vi "MAIN PROGRAM.vi"() -> ()   [LabVIEW 2021]
uses:
  ctlTrialState.ctl
  ctlProtocol.ctl
  ctlProtocolSubID.ctl
  ctlBlockOrder.ctl
  ctrBlockCondition.ctl
  ctrLED_R2L.ctl
  ctrCMCondition.ctl
  ctlSeqFNs.ctl
  ctrBlockInfo.ctl
  ctlBlockInfoSet.ctl
  ctlPkgMain.ctl
  ctlSeqFNs_SubVI PhaseSpace.ctl
  ctlSeqFNs_SubVI ATI.ctl
  ctrOWLMarker.ctl
  ctldistance2plane.ctl
  ctrTrialInfo.ctl
  ctlRecording.ctl
  <vilib>/Analysis/coordinate.llb/Euler Rotation Order.ctl
  <vilib>/DAQmx/write.llb/DAQmx Write (Digital 1D U8 1Chan NSamp).vi
  <vilib>/Analysis/baseanly.llb/A x Vector.vi
  <vilib>/Analysis/baseanly.llb/Real A x B.vi
  <vilib>/Analysis/_algsub.llb/Real Vector Norm.vi
  GLOBAL -MAIN.vi
  <vilib>/DAQmx/miscellaneous.llb/DAQmx Fill In Error Info.vi
  <vilib>/Analysis/Matrix/Numeric/Conversions/Array To Matrix - RA2.vi
  <vilib>/Analysis/Matrix/Numeric/Conversions/Matrix To Array - RM.vi
  <vilib>/Analysis/Matrix/Numeric/Conversions/Array To Matrix - RA.vi
  <vilib>/Analysis/NI_AALBase.lvlib
  <vilib>/Analysis/Matrix/NI_Matrix.lvlib
  <vilib>/Analysis/NI_AALPro.lvlib
panel:
  out "|FM| (N)":dbl format="%#_2g"
  out "|FG| (N)":dbl format="%#_2g"
  out "FM":dbl[](array[numeric]) format="%#_2g"
  out "FG":dbl[](array[numeric]) format="%#.2g"
  out "Roll (deg)":dbl(graph)
  out "Meter":dbl(knob) scale=-15.0..15.0 scale format="%#_2g"
  in  "Time Target (s)":i64=5000
  out "My":dbl
  out "Mx":dbl
  out "friction test?":bool
  out "max roll":dbl
  out "max height":dbl
  in  "BlockInfoSet":T1 {"Trial#-1 in block" min=0 max=11 step=1}
  out "BlockInfoConfig":T2={"block #"=0, "block cond"=enum."RHP", "Trial # in block"=0}
  in  "Subject ID":T4
  out "Current Trial #":i32
  out "Current & finished":T2={"block #"=0, "block cond"=enum."RHP", "Trial # in block"=0}
  out "SYS STATE":T5=enum."INITIALIZE Sub"
  out "CM cond":T6
  out "dCOP (mm)":dbl format="%#_2g"
  out "dCOP cond":T7 items=["all off"=0, "all on"=63, "0 mm"=1, "+8.84 mm"=2, "+15.76 mm"=3, "+22.68 mm"=4, "+29.60 mm"=5, "+36.52 mm"=6, "+43.44 mm"=7, "+50.36 mm"=8, "+57.28 mm"=9, "+64.20 mm"=10, "-8.84 mm"=11, "-15.76 mm"=12, "-22.68 mm"=13, "-29.60 mm"=14, "-36.52 mm"=15, "-43.44 mm"=16, "-50.36 mm"=17, "-57.28 mm"=18, "-64.20 mm"=19]
  out "resultant force":cluster{dbl}(graph)
  out "h (mm)":dbl(graph)
  in  "RepeatTrial":bool
  in  "Recording?":bool=TRUE
  in  "hold criterion (mm)":dbl=50.0 min=0.0 max=500.0 step=1.0
  in  "Path":path=path "C:/Users/NCML/Desktop/GraspEMG/data"
  in  "Bias":bool
  out "ATI":cluster{dbl[][]}[](array[cluster]) {"?" format="%#.2f"}
  out "Protocol":T8={"Subject ID"=enum."sub-09", "Block order"=[enum."famDrop", enum."preDrop", enum."famTask", enum."UL", enum."UR", enum."RHP", enum."LHP", enum."RHD", enum."RLD", enum."LLD", enum."LHD", enum."pstDrop"]}
  out "state":T10
  in  "STOP":bool
  in  "Ready":bool
  out "Date & Time":timestamp format="%<%.3X %x>T"
  # "Recieves data from both SubVIs"
  # "(CCW -; CW +)"
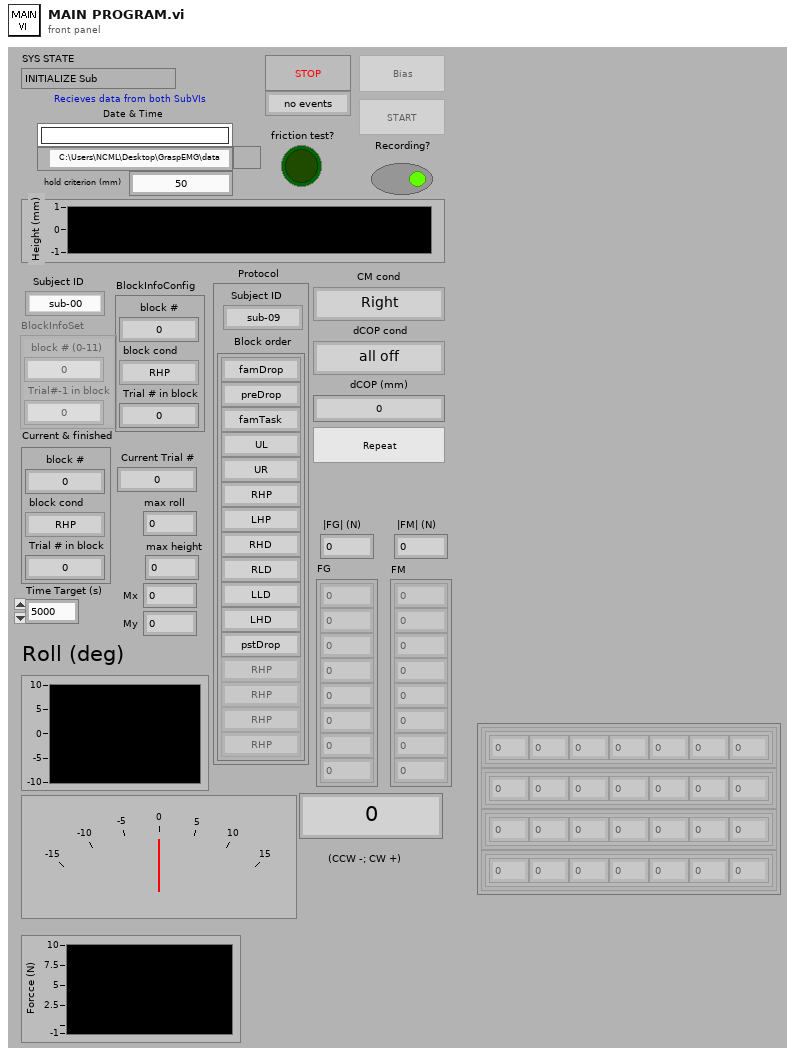
[diagram p1: front panel]
types:
  T1 = typedef "ctlBlockInfoSet.ctl" = cluster{"block # (0-11)":i32, "Trial#-1 in block":i32}
  T2 = typedef "ctrBlockInfo.ctl" = cluster{"block #":i32, "block cond":T3, "Trial # in block":i32}
  T3 = typedef "ctrBlockCondition.ctl" = enum16{"famDrop", "preDrop", "famTask", "RHP", "RLD", "RHD", "LHP", "LLD", "LHD", "UR", "UL", "pstDrop"}
  T4 = typedef "ctlProtocolSubID.ctl" = enum16{"sub-00", "sub-01", "sub-02", "sub-03", "sub-04", "sub-05", "sub-06", "sub-07", "sub-08", "sub-09", "sub-10", "sub-11", "sub-12", "sub-13", "sub-14", "sub-15", "sub-16", "sub-17", "sub-18", "sub-19", "sub-20", "sub-21", "sub-22", "sub-23", "sub-24", "sub-25", "sub-26", "sub-27", "sub-28", "sub-29", "sub-30", "sub-31", "sub-32", "sub-33", "sub-34", "sub-35", "sub-36", "sub-37", "sub-38", "sub-39", "sub-40"}
  T5 = typedef "ctlSeqFNs.ctl" = enum16{"INITIALIZE MAIN", "UpdateProtocol", "UpdateBlockInfo", "UpdatePath", "INITIALIZE Sub", "IDLE", "Bias", "Ready", "RepeatTrial", "Events", "Get PS bias", "Get PhaseSpace", "Get ATI", "Finish", "End PhaseSpace", "End ATI", "ERROR", "EXIT"}
  T6 = typedef "ctrCMCondition.ctl" = enum16{"Right", "Center", "Left"}
  T7 = typedef "ctrLED_R2L.ctl" = u16
  T8 = typedef "ctlProtocol.ctl" = cluster{"Subject ID":T4, "Block order":T9}
  T9 = typedef "ctlBlockOrder.ctl" = T3[]
  T10 = typedef "ctlTrialState.ctl" = enum16{"no events", "ready", "start", "hold", "stop", "end"}
  T11 = typedef "ctlPkgMain.ctl" = cluster{"VIRefNm ":refnum<vi>, "PhaseSpace":refnum<queue>, "ATI":refnum<queue>, "Handle Height":dbl, "Results":cluster{"Kc":string, "Cfg":dbl[]}, "CurrPath":path, "state":T10, "tick ini":i64, "Protocol":T8, "PhaseSpace end?":bool, "ATI end?":bool, "Markers":T12[], "ATI Data":cluster{dbl[][]}[], "d2plane":T13, "data Path":path, "PreTrialInfo":T14, "tdms data":refnum<k34>, "Recording?":bool, "dCOP cond":T7, "TrialInfo":T14, "Handle Tilt":dbl, "maxheight":dbl, "maxroll":dbl, "friction test?":bool, "Trigger Task":refnum<k21>}
  T12 = typedef "ctrOWLMarker.ctl" = cluster{"id":i32, "frame":i32, "x":sgl, "y":sgl, "z":sgl, "cond":sgl, "flag":u32}
  T13 = typedef "ctldistance2plane.ctl" = cluster{"frame":dbl[][]}
  T14 = typedef "ctrTrialInfo.ctl" = cluster{"BlockInfo":T2, "Trial #":i32}
  T15 = enum8{"Enabled", "Disabled", "Disabled and Grayed Out"}
  T16 = enum16{"ALIGN -CENTER", "ALIGN -TOP LEFT", "ALIGN -AS IS", "ALIGN -CUSTOM"}
  T17 = enum16{"open", "open or create", "create or replace", "create", "open (read-only)"}
  T18 = typedef "ctlSeqFNs_SubVI ATI.ctl" = enum16{"INITIALIZE", "SET HANDLE", "IDLE", "READY", "SEND2MAIN", "CALIB Load", "BIAS", "TRIGGER", "END", "ERROR", "EXIT"}
  T19 = typedef "ctlSeqFNs_SubVI PhaseSpace.ctl" = enum16{"INITIALIZE", "IDLE", "BIAS", "READY", "SEND2MAIN", "LOG2TDMS", "TRIGGER", "END", "ERROR", "EXIT"}
  T20 = typedef "ctlRecording.ctl" = cluster{"recording?":bool, "tdms file":refnum<k34>}
  T21 = typedef "NI_AALPro.lvlib/Euler Rotation Order.ctl" = u16
  T22 = typedef "NI_Matrix.lvlib/RealMatrix.ctl" = dbl[][]
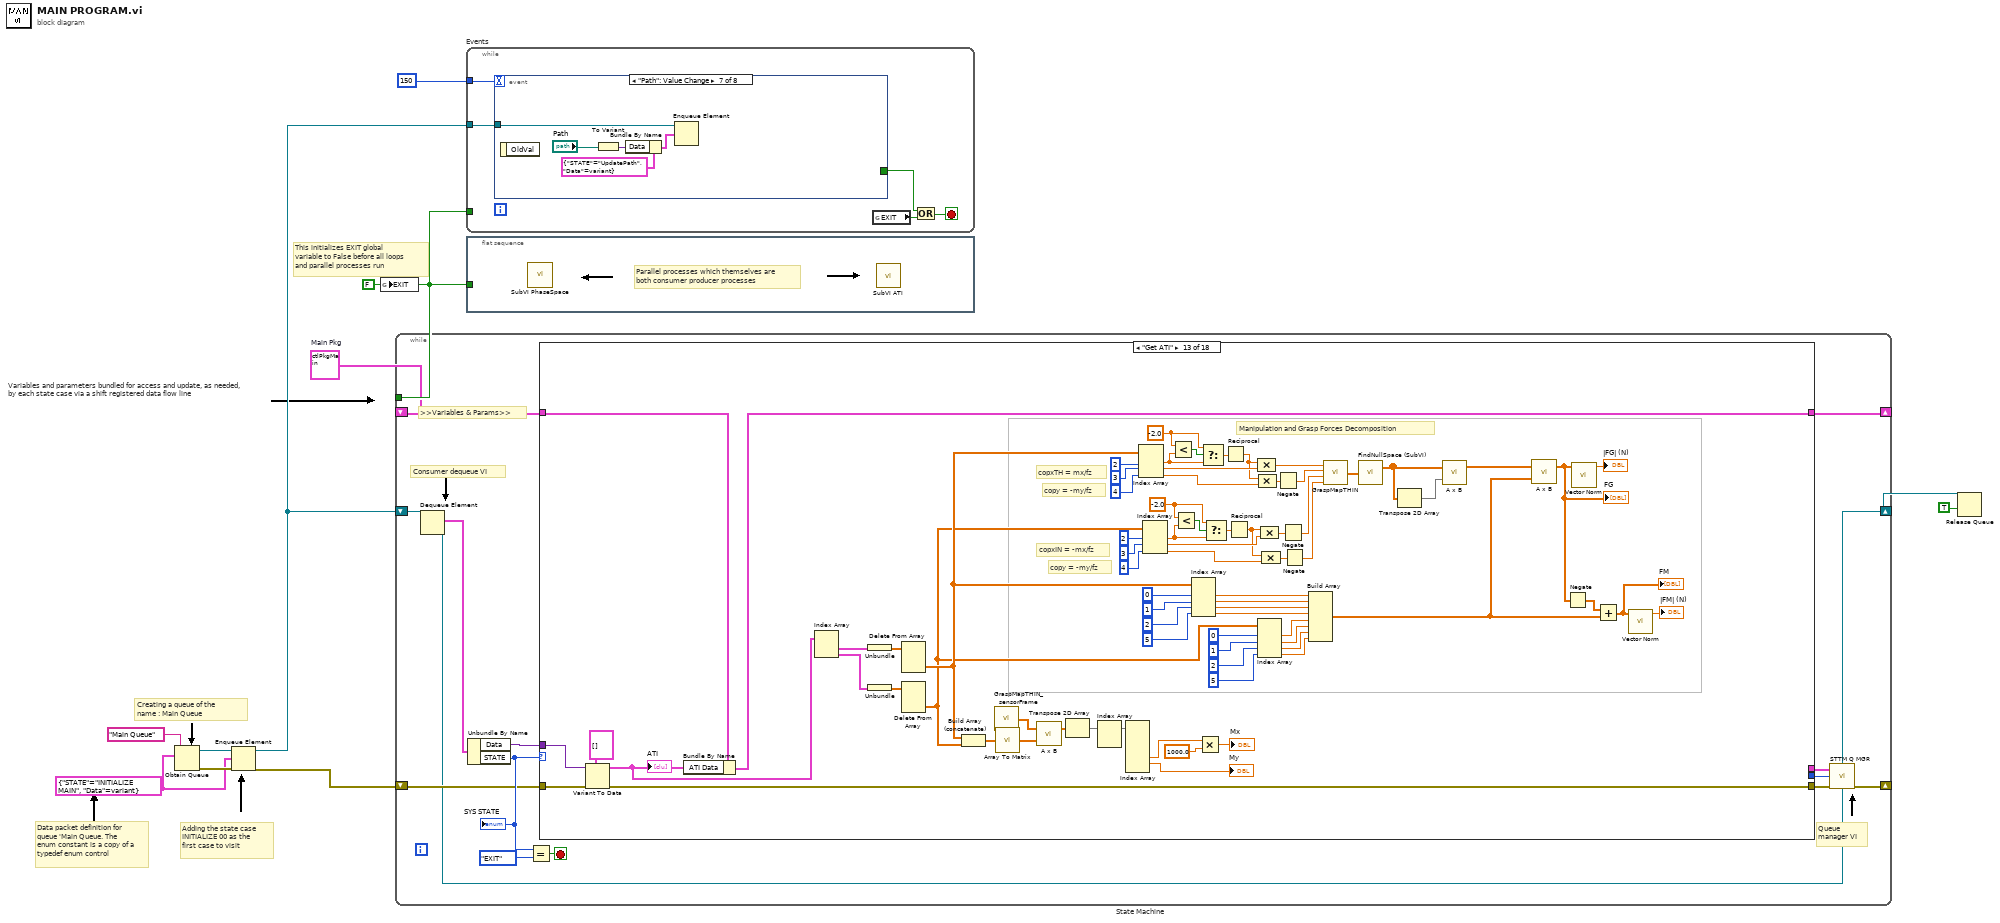
[diagram p0: block diagram]
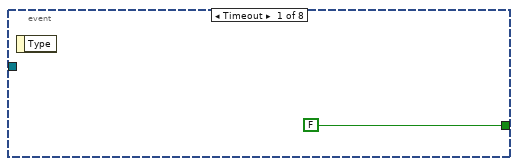
[diagram p2: hidden frame]
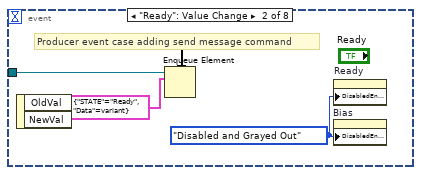
[diagram p3: hidden frame]
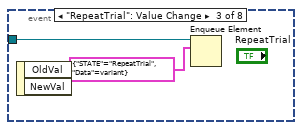
[diagram p4: hidden frame]
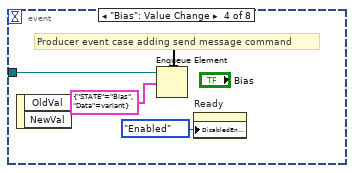
[diagram p5: hidden frame]
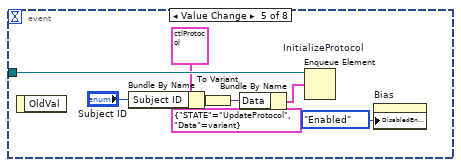
[diagram p6: hidden frame]
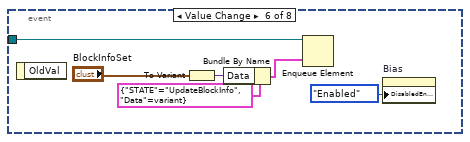
[diagram p7: hidden frame]
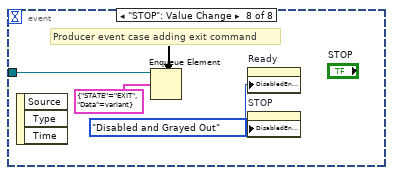
[diagram p8: hidden frame]
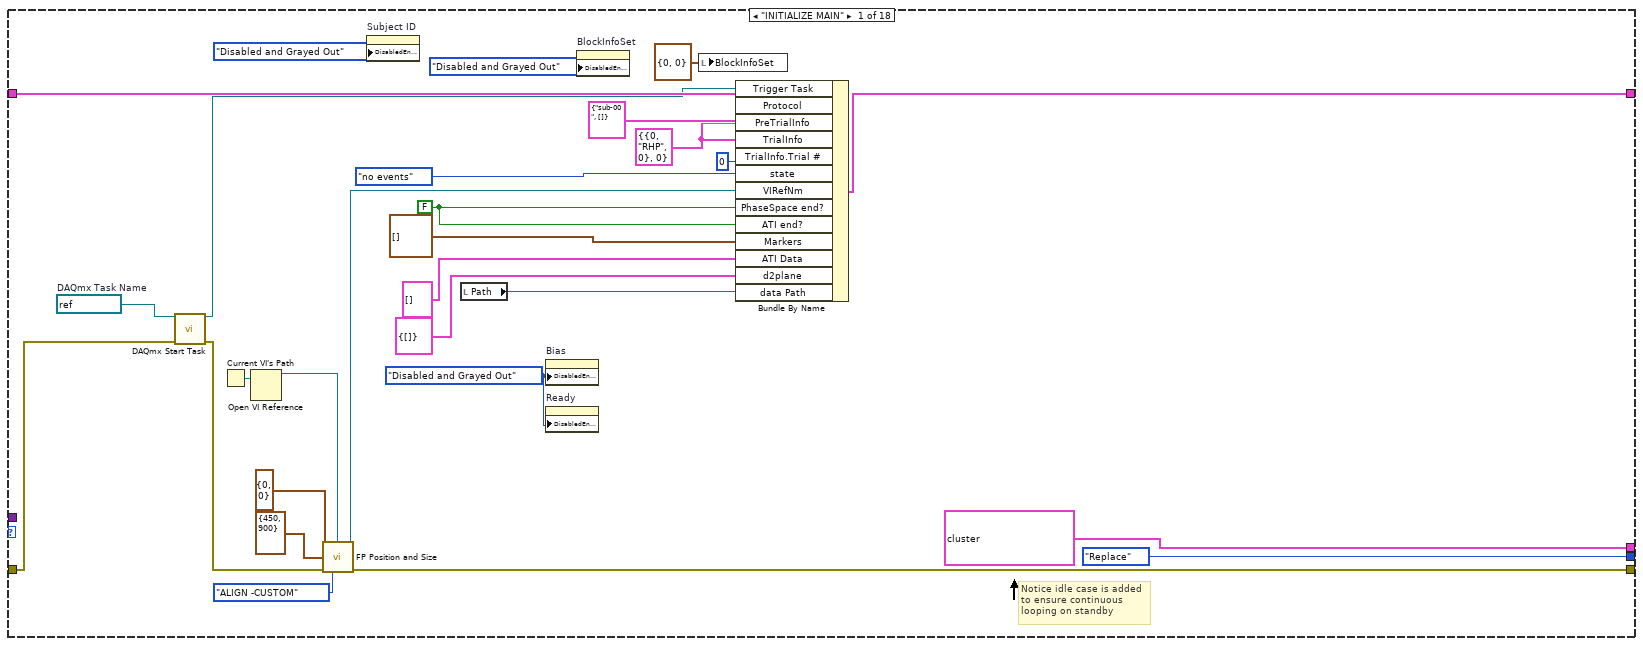
[diagram p9: hidden frame]
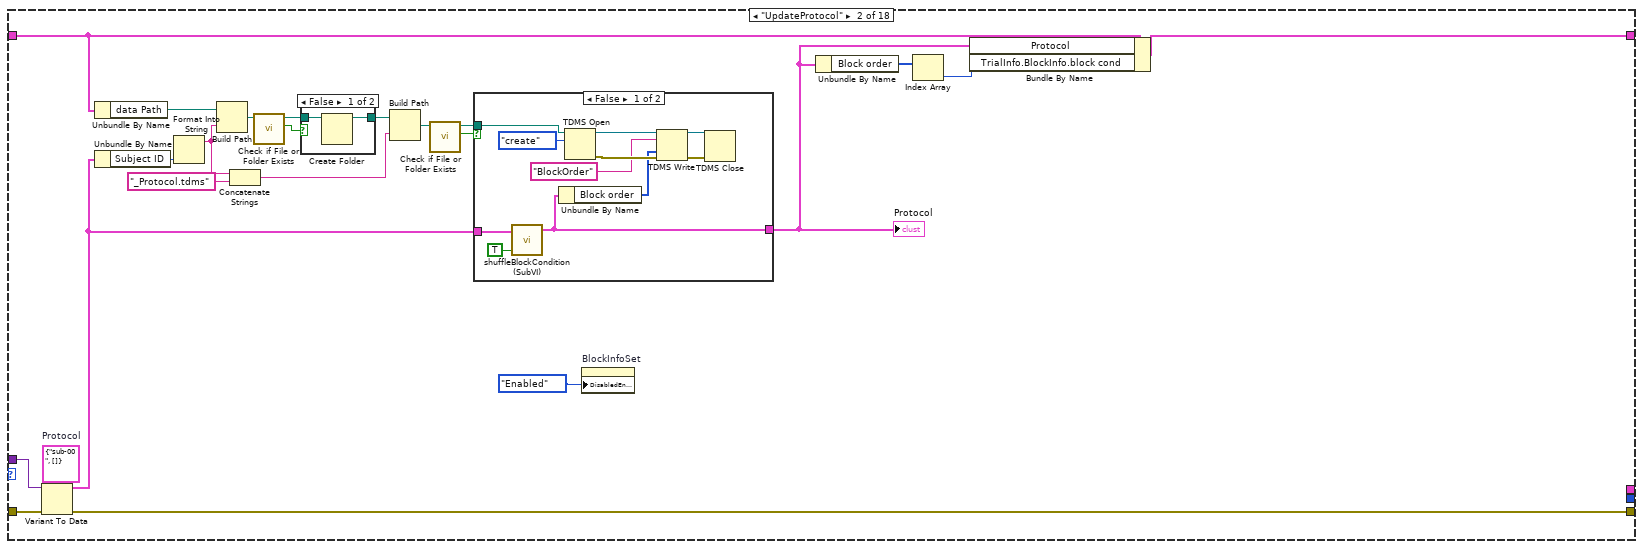
[diagram p10: hidden frame]
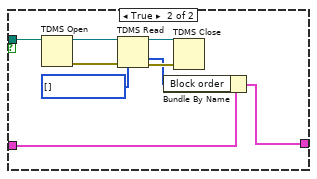
[diagram p12: hidden frame]
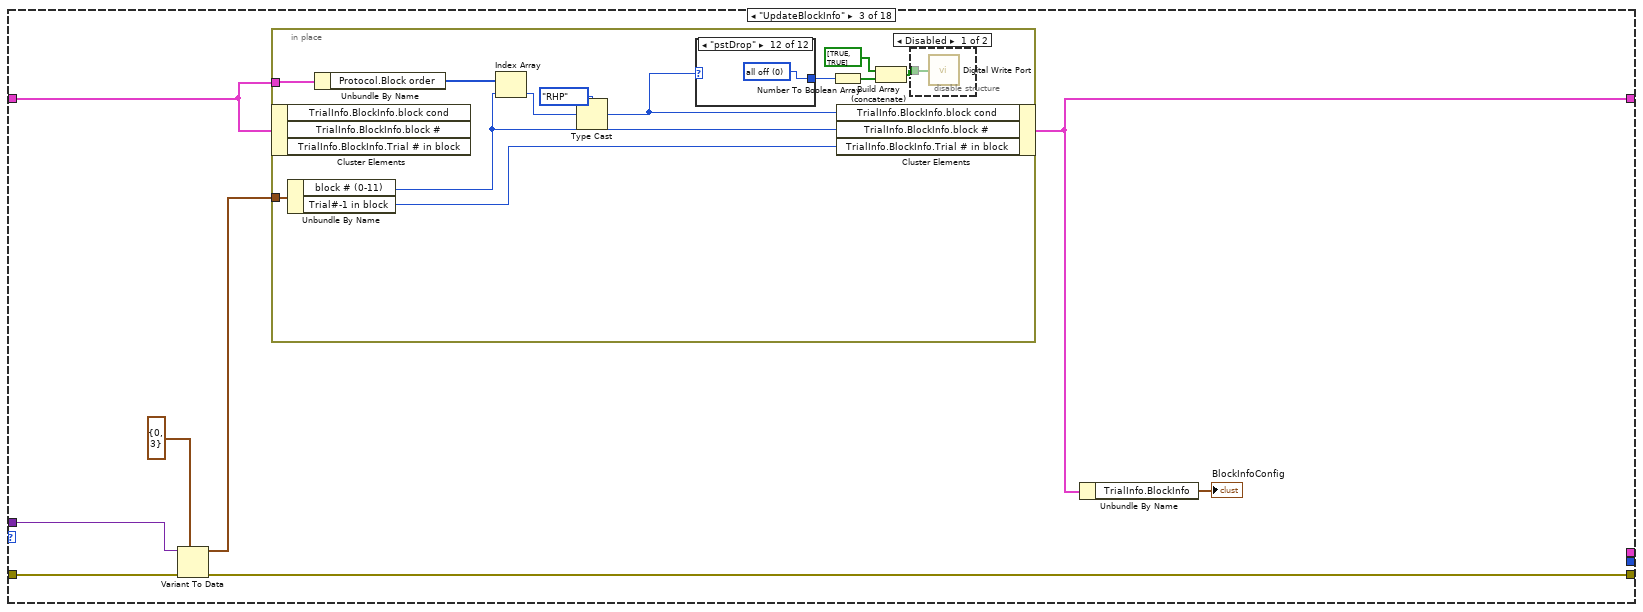
[diagram p13: hidden frame]
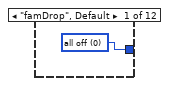
[diagram p15: hidden frame]
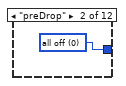
[diagram p16: hidden frame]
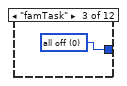
[diagram p17: hidden frame]
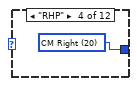
[diagram p18: hidden frame]
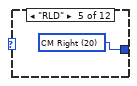
[diagram p19: hidden frame]
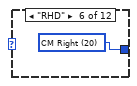
[diagram p20: hidden frame]
diagram:
  w1 = T11 {"VIRefNm "=refnum, "PhaseSpace"=refnum, "ATI"=refnum, "Handle Height"=0.0, "Results"={"Kc"="", "Cfg"=[]}, "CurrPath"=path "", "state"=enum."no events", "tick ini"=0, "Protocol"={"Subject ID"=enum."sub-00", "Block order"=[]}, "PhaseSpace end?"=FALSE, "ATI end?"=FALSE, "Markers"=[], "ATI Data"=[], "d2plane"={"frame"=[]}, "data Path"=path "", "PreTrialInfo"={"BlockInfo"={"block #"=0, "block cond"=enum."RHP", "Trial # in block"=0}, "Trial #"=0}, "tdms data"=refnum, "Recording?"=FALSE, "dCOP cond"=0, "TrialInfo"={"BlockInfo"={"block #"=0, "block cond"=enum."RHP", "Trial # in block"=0}, "Trial #"=0}, "Handle Tilt"=0.0, "maxheight"=0.0, "maxroll"=0.0, "friction test?"=FALSE, "Trigger Task"=""}  # Main Pkg
  w4 = FALSE
  w5 = cluster{"STATE":T5, "Data":variant} {"STATE"=enum."INITIALIZE MAIN", "Data"=variant} ("element")
  # "This initializes EXIT global variable to False before all loops and parallel processes run"
  # "Data packet definition for queue 'Main Queue. The enum constant is a copy of a typedef enum control"
  # "Adding the state case INITIALIZE 00 as the first case to visit"
  # "Creating a queue of the name : Main Queue"
  # "Variables and parameters bundled for access and update, as needed,  by each state case via a shift registered data flow line"
  n1 = Obtain Queue(name (unnamed)="Main Queue" ("Queue Name"), element data type=w5) -> (queue out=w3:refnum<queue>, error out=w7:errorcluster)  [unwired: 3 in, 1 out]
  n2 = Enqueue Element(queue=w3, element=w5, error in (no error)=w7) -> (queue out=w2:refnum<queue>, error out=w6:errorcluster)  [unwired: 1 in, 1 out]
  n3 = global write "GLOBAL -MAIN.vi" "EXIT"(w4) -> ()
  n4 = while "State Machine" {
    shift-right: [w19] -> _
    shift-left: w6 -> [w18]
    shift-right: [w12] -> w9
    shift-left: w2 -> [w25]
    tunnel: w4 -> [_]
    shift-right: [w15] -> _
    shift-left: w1 -> [w16]
    stop <- w17 stop-if-true
    # "Queue manager VI"
    # "Consumer dequeue VI"
    # ">>Variables & Params>>"
    n5 = Dequeue Element(queue=w25) -> (queue out=w12:refnum<queue>, element=w24:cluster{"STATE":T5, "Data":variant})  [unwired: 2 in, 2 out]
    n6 = Unbundle By Name(w24) -> ("Data"=w23:variant, "STATE"=w22:T5)
    "SYS STATE" <- w22
    n7 = Equal?(x=w22, y=ctlSeqFNs."EXIT" ("FN")) -> (x = y?=w17:bool)
    n8 = case shown="\"Get ATI\"" w22 {
      tunnel: w18 -> [w27 w75 w106 w136 w143 w168 w362 w405 w412 w424 w508 w516 w592 w608 w613 w617 w621 w625]
      tunnel: [w36 w76 w107 w137 w141 w167 w360 w402 w412 w432 w507 w515 w591 w598 w613 w617 w620 w627] -> w20
      tunnel: w23 -> [_ w74 w105 w135 _ _ _ _ _ _ w510 w517 w593 _ _ _ _ _]
      tunnel: [cluster{"FN":T5, "Data":variant}[] [{"FN"=enum."INITIALIZE Sub", "Data"=variant}, {"FN"=enum."IDLE", "Data"=variant}] _ _ _ _ w173 _ cluster{"FN":T5, "Data":variant}[] [{"FN"=enum."Events", "Data"=variant}] _ _ _ _ _ _ _ _ _ _] -> w13
      tunnel: w16 -> [w43 w65 w103 w139 w152 w154 w355 w364 w410 w413 w487 w514 w589 w599 w615 w619 w622 w632]
      tunnel: [w48 w66 w102 w138 w151 w165 w354 w403 w411 w413 w506 w513 w588 w597 w614 w618 w622 w632] -> w15
      tunnel: [enum16{"Back", "Front", "Replace"}."Replace" ("FNs") _ _ _ _ enum16{"Back", "Front", "Replace"}."Back" ("FNs") _ enum16{"Back", "Front", "Replace"}."Front" ("FNs") _ _ _ _ _ _ _ _ _ _] -> w14
      frame "INITIALIZE MAIN" {
        w29 = refnum<k21> "Trigger"  # DAQmx Task Name
        w33 = T14 {"BlockInfo"={"block #"=0, "block cond"=enum."RHP", "Trial # in block"=0}, "Trial #"=0} ("PreTrialInfo")
        w38 = T15."Disabled and Grayed Out" ("Disabled")
        w37 = FALSE ("PhaseSpace end?")
        # "Notice idle case is added to ensure continuous looping on standby"
        n9 = call <vilib>:"DAQmx Start Task.vi"("task/channels in"=w29, "error in"=w27) -> ("task out"=w28:refnum<k21>, "error out"=w26:errorcluster)  [unwired: 12 in]
        n10 = Current VI's Path() -> (path=w49:path)
        n11 = Open VI Reference(vi path=w49) -> (vi reference=w50:refnum<vi>)  [unwired: 5 in, 1 out]
        n12 = call "FP Position and Size.vi"("VIRefNum  IN"=w50, "Poistion"=cluster{"left":i16, "top":i16} {"left"=0, "top"=0}, "Size"=cluster{"right":i16, "bottom":i16} {"right"=450, "bottom"=900}, "error in (no error)"=w26, "Mode"=T16."ALIGN -CUSTOM") -> ("VIRefNum OUT"=w47:refnum<vi>, "error out"=w36:errorcluster)  [unwired: 9 in]
        n13 = property on="Subject ID" class="Enum (strict)"("DisabledEnum"=T15."Disabled and Grayed Out" ("Disabled")) -> ()  [unwired: 2 in, 2 out]
        n14 = local read "Path"() -> (w39:path)
        n15 = property on="Bias" class="Bool"("DisabledEnum"=w38) -> ()  [unwired: 2 in, 2 out]
        n16 = property on="Ready" class="Bool"("DisabledEnum"=w38) -> ()  [unwired: 2 in, 2 out]
        n17 = property on="BlockInfoSet" class="Clust (strict)"("DisabledEnum"=T15."Disabled and Grayed Out" ("Disabled")) -> ()  [unwired: 2 in, 2 out]
        n18 = local write "BlockInfoSet"(T1 {"block # (0-11)"=0, "Trial#-1 in block"=0} ("BlockInfoSet")) -> ()
        n19 = Bundle By Name(cluster=w43, "Trigger Task"=w28, "Protocol"=T8 {"Subject ID"=enum."sub-00", "Block order"=[]}, "PreTrialInfo"=w33, "TrialInfo"=w33, "TrialInfo.Trial #"=0 ("Trial #"), "state"=ctlTrialState."no events", "VIRefNm"=w47, "PhaseSpace end?"=w37, "ATI end?"=w37, "Markers"=T12[] [], "ATI Data"=cluster{dbl[][]}[] [] ("Data"), "d2plane"=T13 {"frame"=[]}, "data Path"=w39) -> (w48:T11)
      }
      frame "UpdateProtocol" {
        w73 = T8 {"Subject ID"=enum."sub-00", "Block order"=[]}  # Protocol
        n20 = Variant To Data(error in=w75, type=w73, Variant=w74) -> (data=w67:T8, error out=w76:errorcluster)
        n21 = Unbundle By Name(w65) -> ("data Path"=w62:path)
        n22 = Unbundle By Name(w67) -> ("Subject ID"=w72:T4)
        n23 = Format Into String(w72) -> (resulting string=w63:string)  [unwired: 3 in, 1 out]
        n24 = Build Path(base path=w62, name or relative path=w63) -> (appended path=w61:path)
        n25 = Concatenate Strings(w63, "_Protocol.tdms") -> (w70:string)
        n26 = call <vilib>:"Check if File or Folder Exists.vi"("path"=w61) -> ("file or folder exists?"=w60:bool, "dup path"=w59:path)  [unwired: 8 in, 1 out]
        n27 = case shown="False" w60 {
          tunnel: w59 -> [w78 w79]
          tunnel: [w77 w79] -> w58
          frame False {
            n28 = Create Folder(path (use dialog)=w78) -> (created path=w77:path)  [unwired: 2 in, 2 out]
          }
          frame True {
          }
        }
        n29 = Build Path(base path=w58, name or relative path=w70) -> (appended path=w69:path)
        n30 = call <vilib>:"Check if File or Folder Exists.vi"("path"=w69) -> ("file or folder exists?"=w68:bool, "dup path"=w64:path)  [unwired: 8 in, 1 out]
        n31 = case shown="False" w68 {
          tunnel: w67 -> [w89 w92]
          tunnel: [w88 w91] -> w57
          tunnel: w64 -> [w81 w95]
          frame False {
            n32 = call "shuffleBlockCondition (SubVI).vi"("randomize?(no:F)"=TRUE, "Protocol in"=w89) -> ("Protocol out"=w88:T8)  [unwired: 3 in]
            n33 = Unbundle By Name(w88) -> ("Block order"=w83:T9)
            n34 = TDMS Open(10:T17."create" ("operation (0:open)"), 11:w81) -> (0:w85:errorcluster, 3:w87:refnum<k34>)  [unwired: 5 in]
            n35 = TDMS Write(0:w87, 5:"BlockOrder" ("group name in (Untitled)"), 9:w83, 11:w85) -> (4:w86:refnum<k34>, 15:w84:errorcluster)  [unwired: 2 in, 2 out]
            n36 = TDMS Close(8:w84, 11:w86) -> ()  [unwired: 2 out]
          }
          frame True {
            w94 = T9 [] items=["famDrop", "preDrop", "famTask", "RHP", "RLD", "RHD", "LHP", "LLD", "LHD", "UR", "UL", "pstDrop"] ("Block order")
            n37 = TDMS Open(11:w95) -> (0:w97:errorcluster, 3:w99:refnum<k34>)  [unwired: 6 in]
            n38 = TDMS Read(0:w99, 11:w97, 12:w94) -> (4:w98:refnum<k34>, 10:w93:T9, 15:w96:errorcluster)  [unwired: 5 in, 3 out]
            n39 = Bundle By Name(cluster=w92, "Block order"=w93) -> (w91:T8)
            n40 = TDMS Close(8:w96, 11:w98) -> ()  [unwired: 2 out]
          }
        }
        "Protocol" <- w57
        n41 = property on="BlockInfoSet" class="Clust (strict)"("DisabledEnum"=T15."Enabled" ("Disabled")) -> ()  [unwired: 2 in, 2 out]
        n42 = Unbundle By Name(w57) -> ("Block order"=w56:T9)
        n43 = Index Array(array=w56) -> (element=w55:T3)  [unwired: 1 in]
        n44 = Bundle By Name(cluster=w65, "Protocol"=w57, "TrialInfo.BlockInfo.block cond"=w55) -> (w66:T11)
      }
      frame "UpdateBlockInfo" {
        n45 = Variant To Data(error in=w106, type=T1 {"block # (0-11)"=0, "Trial#-1 in block"=3} ("BlockInfoSet"), Variant=w105) -> (data=w104:T1, error out=w107:errorcluster)
        n46 = in-place {
          in-place-border: w103 -> [w119]
          in-place-border: w104 -> [w117]
          n47 = in-place-cluster #1(w103) -> ()  [unwired: 3 out]
          n48 = Unbundle By Name(w117) -> ("block # (0-11)"=w116:i32, "Trial#-1 in block"=w115:i32)
          n49 = Unbundle By Name(w119) -> ("Protocol.Block order"=w118:T9)
          n50 = Index Array(array=w118, index=w116) -> (element=w114:T3)
          n51 = Type Cast(type=ctrBlockCondition."RHP" ("TrialInfo.BlockInfo.block cond"), x=w114) -> (*(type *) &x=w108:T3)
          n52 = case shown="\"pstDrop\"" w108 {
            tunnel: [w121 w122 w123 w124 w125 w126 w127 w128 w129 w130 w131 w132] -> w110
            frame "famDrop", Default {
              w121 = T7 0 items=["all off"=0, "all on"=63, "0 mm"=1, "+8.84 mm"=2, "+15.76 mm"=3, "+22.68 mm"=4, "+29.60 mm"=5, "+36.52 mm"=6, "+43.44 mm"=7, "+50.36 mm"=8, "+57.28 mm"=9, "+64.20 mm"=10, "-8.84 mm"=11, "-15.76 mm"=12, "-22.68 mm"=13, "-29.60 mm"=14, "-36.52 mm"=15, "-43.44 mm"=16, "-50.36 mm"=17, "-57.28 mm"=18, "-64.20 mm"=19, "CM Right"=20, "CM Left"=21] ("dCOP cond 2")
            }
            frame "preDrop" {
              w122 = T7 0 items=["all off"=0, "all on"=63, "0 mm"=1, "+8.84 mm"=2, "+15.76 mm"=3, "+22.68 mm"=4, "+29.60 mm"=5, "+36.52 mm"=6, "+43.44 mm"=7, "+50.36 mm"=8, "+57.28 mm"=9, "+64.20 mm"=10, "-8.84 mm"=11, "-15.76 mm"=12, "-22.68 mm"=13, "-29.60 mm"=14, "-36.52 mm"=15, "-43.44 mm"=16, "-50.36 mm"=17, "-57.28 mm"=18, "-64.20 mm"=19, "CM Right"=20, "CM Left"=21] ("dCOP cond 2")
            }
            frame "famTask" {
              w123 = T7 0 items=["all off"=0, "all on"=63, "0 mm"=1, "+8.84 mm"=2, "+15.76 mm"=3, "+22.68 mm"=4, "+29.60 mm"=5, "+36.52 mm"=6, "+43.44 mm"=7, "+50.36 mm"=8, "+57.28 mm"=9, "+64.20 mm"=10, "-8.84 mm"=11, "-15.76 mm"=12, "-22.68 mm"=13, "-29.60 mm"=14, "-36.52 mm"=15, "-43.44 mm"=16, "-50.36 mm"=17, "-57.28 mm"=18, "-64.20 mm"=19, "CM Right"=20, "CM Left"=21] ("dCOP cond 2")
            }
            frame "RHP" {
              w124 = T7 20 items=["all off"=0, "all on"=63, "0 mm"=1, "+8.84 mm"=2, "+15.76 mm"=3, "+22.68 mm"=4, "+29.60 mm"=5, "+36.52 mm"=6, "+43.44 mm"=7, "+50.36 mm"=8, "+57.28 mm"=9, "+64.20 mm"=10, "-8.84 mm"=11, "-15.76 mm"=12, "-22.68 mm"=13, "-29.60 mm"=14, "-36.52 mm"=15, "-43.44 mm"=16, "-50.36 mm"=17, "-57.28 mm"=18, "-64.20 mm"=19, "CM Right"=20, "CM Left"=21] ("dCOP cond 2")
            }
            frame "RLD" {
              w125 = T7 20 items=["all off"=0, "all on"=63, "0 mm"=1, "+8.84 mm"=2, "+15.76 mm"=3, "+22.68 mm"=4, "+29.60 mm"=5, "+36.52 mm"=6, "+43.44 mm"=7, "+50.36 mm"=8, "+57.28 mm"=9, "+64.20 mm"=10, "-8.84 mm"=11, "-15.76 mm"=12, "-22.68 mm"=13, "-29.60 mm"=14, "-36.52 mm"=15, "-43.44 mm"=16, "-50.36 mm"=17, "-57.28 mm"=18, "-64.20 mm"=19, "CM Right"=20, "CM Left"=21] ("dCOP cond 2")
            }
            frame "RHD" {
              w126 = T7 20 items=["all off"=0, "all on"=63, "0 mm"=1, "+8.84 mm"=2, "+15.76 mm"=3, "+22.68 mm"=4, "+29.60 mm"=5, "+36.52 mm"=6, "+43.44 mm"=7, "+50.36 mm"=8, "+57.28 mm"=9, "+64.20 mm"=10, "-8.84 mm"=11, "-15.76 mm"=12, "-22.68 mm"=13, "-29.60 mm"=14, "-36.52 mm"=15, "-43.44 mm"=16, "-50.36 mm"=17, "-57.28 mm"=18, "-64.20 mm"=19, "CM Right"=20, "CM Left"=21] ("dCOP cond 2")
            }
            frame "LHP" {
              w127 = T7 21 items=["all off"=0, "all on"=63, "0 mm"=1, "+8.84 mm"=2, "+15.76 mm"=3, "+22.68 mm"=4, "+29.60 mm"=5, "+36.52 mm"=6, "+43.44 mm"=7, "+50.36 mm"=8, "+57.28 mm"=9, "+64.20 mm"=10, "-8.84 mm"=11, "-15.76 mm"=12, "-22.68 mm"=13, "-29.60 mm"=14, "-36.52 mm"=15, "-43.44 mm"=16, "-50.36 mm"=17, "-57.28 mm"=18, "-64.20 mm"=19, "CM Right"=20, "CM Left"=21] ("dCOP cond 2")
            }
            frame "LLD" {
              w128 = T7 21 items=["all off"=0, "all on"=63, "0 mm"=1, "+8.84 mm"=2, "+15.76 mm"=3, "+22.68 mm"=4, "+29.60 mm"=5, "+36.52 mm"=6, "+43.44 mm"=7, "+50.36 mm"=8, "+57.28 mm"=9, "+64.20 mm"=10, "-8.84 mm"=11, "-15.76 mm"=12, "-22.68 mm"=13, "-29.60 mm"=14, "-36.52 mm"=15, "-43.44 mm"=16, "-50.36 mm"=17, "-57.28 mm"=18, "-64.20 mm"=19, "CM Right"=20, "CM Left"=21] ("dCOP cond 2")
            }
            frame "LHD" {
              w129 = T7 21 items=["all off"=0, "all on"=63, "0 mm"=1, "+8.84 mm"=2, "+15.76 mm"=3, "+22.68 mm"=4, "+29.60 mm"=5, "+36.52 mm"=6, "+43.44 mm"=7, "+50.36 mm"=8, "+57.28 mm"=9, "+64.20 mm"=10, "-8.84 mm"=11, "-15.76 mm"=12, "-22.68 mm"=13, "-29.60 mm"=14, "-36.52 mm"=15, "-43.44 mm"=16, "-50.36 mm"=17, "-57.28 mm"=18, "-64.20 mm"=19, "CM Right"=20, "CM Left"=21] ("dCOP cond 2")
            }
            frame "UR" {
              w130 = T7 20 items=["all off"=0, "all on"=63, "0 mm"=1, "+8.84 mm"=2, "+15.76 mm"=3, "+22.68 mm"=4, "+29.60 mm"=5, "+36.52 mm"=6, "+43.44 mm"=7, "+50.36 mm"=8, "+57.28 mm"=9, "+64.20 mm"=10, "-8.84 mm"=11, "-15.76 mm"=12, "-22.68 mm"=13, "-29.60 mm"=14, "-36.52 mm"=15, "-43.44 mm"=16, "-50.36 mm"=17, "-57.28 mm"=18, "-64.20 mm"=19, "CM Right"=20, "CM Left"=21] ("dCOP cond 2")
            }
            frame "UL" {
              w131 = T7 21 items=["all off"=0, "all on"=63, "0 mm"=1, "+8.84 mm"=2, "+15.76 mm"=3, "+22.68 mm"=4, "+29.60 mm"=5, "+36.52 mm"=6, "+43.44 mm"=7, "+50.36 mm"=8, "+57.28 mm"=9, "+64.20 mm"=10, "-8.84 mm"=11, "-15.76 mm"=12, "-22.68 mm"=13, "-29.60 mm"=14, "-36.52 mm"=15, "-43.44 mm"=16, "-50.36 mm"=17, "-57.28 mm"=18, "-64.20 mm"=19, "CM Right"=20, "CM Left"=21] ("dCOP cond 2")
            }
            frame "pstDrop" {
              w132 = T7 0 items=["all off"=0, "all on"=63, "0 mm"=1, "+8.84 mm"=2, "+15.76 mm"=3, "+22.68 mm"=4, "+29.60 mm"=5, "+36.52 mm"=6, "+43.44 mm"=7, "+50.36 mm"=8, "+57.28 mm"=9, "+64.20 mm"=10, "-8.84 mm"=11, "-15.76 mm"=12, "-22.68 mm"=13, "-29.60 mm"=14, "-36.52 mm"=15, "-43.44 mm"=16, "-50.36 mm"=17, "-57.28 mm"=18, "-64.20 mm"=19, "CM Right"=20, "CM Left"=21] ("dCOP cond 2")
            }
          }
          n53 = Number To Boolean Array(number=w110) -> (Boolean array=w112:bool[])
          n54 = in-place-cluster #1("TrialInfo.BlockInfo.block cond"=w108, "TrialInfo.BlockInfo.block #"=w116, "TrialInfo.BlockInfo.Trial # in block"=w115) -> (w102:T11)
          n55 = Build Array (concatenate)(bool[] [TRUE, TRUE] ("element"), w112) -> (w109:bool[])
          n56 = disable-structure shown="Disabled" {
            disable-tunnel: w109 -> [w120 _]
            frame Disabled {
              n57 = call <vilib>:"Digital Write Port.vi"("Pin Values"=w120) -> ()  [unwired: 13 in, 2 out]
            }
            frame Enabled {
            }
          }
        }
        n58 = Unbundle By Name(w102) -> ("TrialInfo.BlockInfo"=→"BlockInfoConfig":T2)
      }
      frame "UpdatePath" {
        n59 = Variant To Data(error in=w136, type=path "", Variant=w135) -> (data=w134:path, error out=w137:errorcluster)
        n60 = Bundle By Name(cluster=w139, "data Path"=w134) -> (w138:T11)
      }
      frame "INITIALIZE Sub" {
        # "Queue grabbed for other parallel processes allows sending commands and data to those processes"
        n61 = Obtain Queue(name (unnamed)="PhaseSpace", element data type=cluster{"STATE":T19, "Data":variant} {"STATE"=enum."INITIALIZE", "Data"=variant} ("element"), error in (no error)=w143) -> (queue out=w145:refnum<queue>, error out=w150:errorcluster)  [unwired: 2 in, 1 out]
        n62 = Obtain Queue(name (unnamed)="ATI", element data type=cluster{"STATE":T18, "Data":variant} {"STATE"=enum."INITIALIZE", "Data"=variant} ("element"), error in (no error)=w150) -> (queue out=w144:refnum<queue>, error out=w142:errorcluster)  [unwired: 2 in, 1 out]
        n63 = property on="Subject ID" class="Enum (strict)"(error in=w142, "DisabledEnum"=T15."Enabled" ("Disabled")) -> (error out=w141:errorcluster)  [unwired: 1 in, 1 out]
        n64 = Bundle By Name(cluster=w152, "PhaseSpace"=w145, "ATI"=w144) -> (w151:T11)
      }
      frame "IDLE" {
        # "Idle state case added within the idle case to sustain looping"
        n65 = Unbundle By Name(w154) -> ("ATI Data"=w159:cluster{dbl[][]}[], "PhaseSpace end?"=w161:bool, "ATI end?"=w164:bool, "tdms data"=w169:refnum<k34>)
        n66 = Wait Until Next ms Multiple(millisecond multiple=u32 20) -> ()  [unwired: 1 out]
        n67 = Unbundle By Name(w154) -> ("friction test?"=w153:bool, "tick ini"=w170:i64, "Handle Height"=w175:dbl, "state"=w176:T10)
        "state" <- w176
        n68 = Get Date/Time In Seconds() -> (seconds since 1Jan1904=→"Date & Time":timestamp)
        n69 = Array Size(array=w159) -> (size(s)=w158:i32)
        n70 = And(x=w161, y=w164) -> (x .and. y?=w160:bool)
        n71 = Decrement(x=w158) -> (x-1=w157:i32)
        n72 = Not Equal To 0?(x=w157) -> (x != 0?=w156:bool)
        n73 = case shown="True" w156 {
          tunnel: w159 -> [w322 w345]
          tunnel: [w316 _] -> w155
          frame True {
            w311 = -2.0
            w301 = -2.0
            n74 = Index Array(array=w322) -> (element #1=w324:cluster{dbl[][]}, element #2=w323:cluster{dbl[][]})  [unwired: 2 in]
            n75 = Unbundle(w324) -> (w321:dbl[][])
            n76 = Unbundle(w323) -> (w320:dbl[][])
            n77 = Delete From Array(array=w320) -> (deleted portion=w300:dbl[])  [unwired: 3 in, 1 out]
            n78 = Delete From Array(array=w321) -> (deleted portion=w299:dbl[])  [unwired: 3 in, 1 out]
            n79 = Index Array(array=w299, index #1=2 ("index"), index #2=4 ("index"), index #3=0 ("index")) -> (element #1=w296:dbl, element #2=w317:dbl, element #3=w294:dbl)
            n80 = Index Array(array=w300, index #1=2 ("index"), index #2=4 ("index"), index #3=0 ("index")) -> (element #1=w295:dbl, element #2=w306:dbl, element #3=w293:dbl)
            n81 = Less?(x=w301, y=w296) -> (x < y?=w313:bool)
            n82 = Less?(x=w311, y=w295) -> (x < y?=w310:bool)
            n83 = Add(x=w294, y=w293) -> (x+y=w290:dbl)
            n84 = Select(t=w301, s=w313, f=w296) -> (s? t:f=w314:dbl)
            n85 = Select(t=w311, s=w310, f=w295) -> (s? t:f=w309:dbl)
            n86 = Negate(x=w290) -> (-x=w289:dbl)
            n87 = Reciprocal(x=w314) -> (1/x=w319:dbl)
            n88 = Reciprocal(x=w309) -> (1/x=w307:dbl)
            n89 = Compound Arithmetic op=MULTIPLY(1000.0 ("value"), w319, w317) -> (w304:dbl)
            n90 = Compound Arithmetic op=MULTIPLY(1000.0 ("value"), w307, w306) -> (w305:dbl)
            n91 = Negate(x=w304) -> (-x=w303:dbl)
            n92 = Add(x=w303, y=w305) -> (x+y=→"dCOP (mm)":dbl)
            n93 = Bundle(w289) -> (w316:cluster{dbl})  [unwired: 1 in]
          }
          frame False {
            n94 = Index Array(array=w345) -> (element=w346:cluster{dbl[][]})  [unwired: 1 in]
            n95 = Unbundle(w346) -> (w333:dbl[][])
            n96 = Delete From Array(array=w333) -> (deleted portion=w344:dbl[])  [unwired: 3 in, 1 out]
            n97 = Index Array(array=w344, index #4=6 ("index"), index #5=7 ("index"), index #6=8 ("index")) -> (element #1=w343:dbl, element #2=w342:dbl, element #3=w341:dbl, element #4=w327:dbl, element #5=w326:dbl, element #6=w325:dbl)  [unwired: 3 in]
            n98 = Negate(x=w326) -> (-x=w329:dbl)
            n99 = Negate(x=w325) -> (-x=w328:dbl)
            n100 = Compound Arithmetic op=ADD(w343, w327) -> (w338:dbl)
            n101 = Compound Arithmetic op=ADD(w342, w329) -> (w339:dbl)
            n102 = Compound Arithmetic op=ADD(w341, w328) -> (w340:dbl)
            n103 = Square(x=w338) -> (x^2=w337:dbl)
            n104 = Square(x=w339) -> (x^2=w336:dbl)
            n105 = Square(x=w340) -> (x^2=w335:dbl)
            n106 = Compound Arithmetic op=ADD(w337, w336, w335) -> (w334:dbl)
            n107 = Square Root(x=w334) -> ()  [unwired: 1 out]
          }
        }
        "resultant force" <- w155
        n108 = case shown="True" w160 {
          tunnel: w169 -> [_ w353]
          tunnel: w168 -> [w349 w352]
          tunnel: [w349 w351] -> w167
          tunnel: [w348 w350] -> w163
          tunnel: w161 -> [w348 _]
          tunnel: [w347 w350] -> w162
          tunnel: w164 -> [w347 _]
          frame False {
          }
          frame True {
            w350 = FALSE
            n109 = TDMS Close(8:w352, 11:w353) -> (0:w351:errorcluster)  [unwired: 1 out]
          }
        }
        n110 = case shown="True" w153 {
          tunnel: w176 -> [w184 w256]
          tunnel: w175 -> [w183 w255]
          tunnel: [w182 w254] -> w171
          tunnel: w170 -> [w181 w253]
          tunnel: [w180 w252] -> w166
          tunnel: w154 -> [w179 w251]
          frame False {
            n111 = case shown="\"hold\"" w184 {
              tunnel: w183 -> [_ _ w205 _ _]
              tunnel: w179 -> [w185 w194 w208 w218 w242]
              tunnel: [w185 w193 w207 w225 w241] -> w180
              tunnel: [_ w192 w204 w224 w240] -> w182
              tunnel: w181 -> [_ w190 _ w220 w235]
              frame "no events", Default {
              }
              frame "ready" {
                n112 = Tick Count (ms)() -> (millisecond timer value=w191:u32)
                n113 = To Quad Integer(1:w191) -> (0:w189:i64)
                n114 = Add(x=w190, y=w189) -> (x+y=w187:i64)
                n115 = Less?(x=i64 1500 ("Time Target (s)"), y=w187) -> (x < y?=w188:bool)
                n116 = case shown="True" w188 {
                  tunnel: w194 -> [w195 w202]
                  tunnel: [w195 w201] -> w193
                  tunnel: [_ cluster{"FN":T5, "Data":variant}[] [{"FN"=enum."Events", "Data"=variant}]] -> w192
                  frame False {
                  }
                  frame True {
                    n117 = Tick Count (ms)() -> (millisecond timer value=w197:u32)
                    n118 = To Quad Integer(1:w197) -> (0:w198:i64)
                    n119 = Negate(x=w198) -> (-x=w196:i64)
                    n120 = Bundle By Name(cluster=w202, "state"=ctlTrialState."start", "tick ini"=w196) -> (w201:T11)
                  }
                }
              }
              frame "start" {
                n121 = Less?(x="hold criterion (mm)", y=w205) -> (x < y?=w203:bool)
                n122 = case shown="True" w203 {
                  tunnel: w208 -> [w209 w216]
                  tunnel: [w209 w215] -> w207
                  tunnel: [_ cluster{"FN":T5, "Data":variant}[] [{"FN"=enum."Events", "Data"=variant}]] -> w204
                  frame False {
                  }
                  frame True {
                    n123 = Tick Count (ms)() -> (millisecond timer value=w212:u32)
                    n124 = To Quad Integer(1:w212) -> (0:w211:i64)
                    n125 = Negate(x=w211) -> (-x=w210:i64)
                    n126 = Bundle By Name(cluster=w216, "state"=ctlTrialState."hold", "tick ini"=w210) -> (w215:T11)
                  }
                }
              }
              frame "hold" {
                n127 = Tick Count (ms)() -> (millisecond timer value=w223:u32)
                n128 = To Quad Integer(1:w223) -> (0:w222:i64)
                n129 = Add(x=w220, y=w222) -> (x+y=w221:i64)
                n130 = Less?(x=i64 2000, y=w221) -> (x < y?=w219:bool)
                n131 = case shown="True" w219 {
                  tunnel: w218 -> [w226 w233]
                  tunnel: [w226 w232] -> w225
                  tunnel: [_ cluster{"FN":T5, "Data":variant}[] [{"FN"=enum."Events", "Data"=variant}]] -> w224
                  frame False {
                  }
                  frame True {
                    n132 = Tick Count (ms)() -> (millisecond timer value=w229:u32)
                    n133 = To Quad Integer(1:w229) -> (0:w228:i64)
                    n134 = Negate(x=w228) -> (-x=w227:i64)
                    n135 = Bundle By Name(cluster=w233, "state"=ctlTrialState."stop", "tick ini"=w227) -> (w232:T11)
                  }
                }
              }
              frame "stop" {
                n136 = Tick Count (ms)() -> (millisecond timer value=w239:u32)
                n137 = To Quad Integer(1:w239) -> (0:w238:i64)
                n138 = Add(x=w235, y=w238) -> (x+y=w237:i64)
                n139 = Less?(x=i64 3000 ("Time Target (s)"), y=w237) -> (x < y?=w234:bool)
                n140 = case shown="True" w234 {
                  tunnel: w242 -> [w243 w250]
                  tunnel: [w243 w249] -> w241
                  tunnel: [_ cluster{"FN":T5, "Data":variant}[] [{"FN"=enum."Events", "Data"=variant}, {"FN"=enum."Finish", "Data"=variant}]] -> w240
                  frame False {
                  }
                  frame True {
                    n141 = Tick Count (ms)() -> (millisecond timer value=w245:u32)
                    n142 = To Quad Integer(1:w245) -> (0:w246:i64)
                    n143 = Negate(x=w246) -> (-x=w244:i64)
                    n144 = Bundle By Name(cluster=w250, "state"=ctlTrialState."end", "tick ini"=w244) -> (w249:T11)
                  }
                }
              }
            }
          }
          frame True {
            n145 = case shown="\"ready\"" w256 {
              tunnel: w255 -> [_ _ w277]
              tunnel: w251 -> [w257 w266 w280]
              tunnel: [w257 w265 w279] -> w252
              tunnel: [_ w264 w276] -> w254
              tunnel: w253 -> [_ w262 _]
              frame "no events", Default {
              }
              frame "ready" {
                n146 = Tick Count (ms)() -> (millisecond timer value=w263:u32)
                n147 = To Quad Integer(1:w263) -> (0:w261:i64)
                n148 = Add(x=w262, y=w261) -> (x+y=w259:i64)
                n149 = Less?(x="Time Target (s)", y=w259) -> (x < y?=w260:bool)
                n150 = case shown="True" w260 {
                  tunnel: w266 -> [w267 w274]
                  tunnel: [w267 w273] -> w265
                  tunnel: [_ cluster{"FN":T5, "Data":variant}[] [{"FN"=enum."Events", "Data"=variant}]] -> w264
                  frame False {
                  }
                  frame True {
                    n151 = Tick Count (ms)() -> (millisecond timer value=w269:u32)
                    n152 = To Quad Integer(1:w269) -> (0:w270:i64)
                    n153 = Negate(x=w270) -> (-x=w268:i64)
                    n154 = Bundle By Name(cluster=w274, "state"=ctlTrialState."start", "tick ini"=w268) -> (w273:T11)
                  }
                }
              }
              frame "start" {
                n155 = Greater?(x=20.0 ("hold criterion (mm) 2"), y=w277) -> (0:w275:bool)
                n156 = case shown="True" w275 {
                  tunnel: w280 -> [w281 w288]
                  tunnel: [w281 w287] -> w279
                  tunnel: [_ cluster{"FN":T5, "Data":variant}[] [{"FN"=enum."Events", "Data"=variant}, {"FN"=enum."Finish", "Data"=variant}]] -> w276
                  frame False {
                  }
                  frame True {
                    n157 = Tick Count (ms)() -> (millisecond timer value=w284:u32)
                    n158 = To Quad Integer(1:w284) -> (0:w283:i64)
                    n159 = Negate(x=w283) -> (-x=w282:i64)
                    n160 = Bundle By Name(cluster=w288, "state"=ctlTrialState."end", "tick ini"=w282) -> (w287:T11)
                  }
                }
              }
            }
          }
        }
        n161 = Bundle By Name(cluster=w166, "PhaseSpace end?"=w163, "ATI end?"=w162) -> (w165:T11)
        n162 = Build Array (concatenate)(w171, cluster{"FN":T5, "Data":variant}[] [{"FN"=enum."IDLE", "Data"=variant}]) -> (w173:cluster{"FN":T5, "Data":variant}[])
      }
      frame "Bias" {
        n163 = Unbundle By Name(w355) -> ("PhaseSpace"=w358:refnum<queue>, "ATI"=w359:refnum<queue>)
        n164 = in-place {
          w363 = 0.0 ("maxdist")
          n165 = in-place-cluster #2(w355) -> ()  [unwired: 2 out]
          n166 = in-place-cluster #2("maxheight"=w363, "maxroll"=w363) -> (w354:T11)
        }
        n167 = Enqueue Element(queue=w359, element=cluster{"STATE":T18, "Data":variant} {"STATE"=enum."BIAS", "Data"=variant}, error in (no error)=w362) -> (error out=w361:errorcluster)  [unwired: 1 in, 2 out]
        n168 = Enqueue Element(queue=w358, element=cluster{"STATE":T19, "Data":variant} {"STATE"=enum."BIAS", "Data"=variant}, error in (no error)=w361) -> (error out=w360:errorcluster)  [unwired: 1 in, 2 out]
      }
      frame "Ready" {
        w369 = T3[] [enum."famDrop", enum."preDrop", enum."pstDrop"] items=["famDrop", "preDrop", "famTask", "RHP", "RLD", "RHD", "LHP", "LLD", "LHD", "UR", "UL", "pstDrop"]
        n169 = Unbundle By Name(w364) -> ("TrialInfo"=w372:T14, "Protocol"=w374:T8, "data Path"=w385:path, "PhaseSpace"=w391:refnum<queue>, "ATI"=w392:refnum<queue>)
        n170 = call "updateTrialInfo (SubVI).vi"("data Path"=w385, "Protocol"=w374, "currentBlockInfo"=w372) -> ("file path out"=w381:path, "dCOP cond"=w375:T7, "CM cond"=→"CM cond":T6, "next"=w370:T14)  [unwired: 1 in]
        "dCOP cond" <- w375
        n171 = Strip Path(path=w381) -> (stripped path=w380:path)  [unwired: 1 out]
        n172 = Unbundle By Name(w370) -> ("Trial #"=→"Current Trial #":i32, "BlockInfo"=→"Current & finished":T2)
        n173 = Build Path(base path=w380, name or relative path="dummy") -> (appended path=w378:path)
        n174 = Select(t=w381, s="Recording?", f=w378) -> (s? t:f=w382:path)
        n175 = Unbundle By Name(w370) -> ("BlockInfo.block cond"=w368:T3)
        n176 = TDMS Open(6:FALSE ("disable buffering? (T)"), 10:T17."create or replace" ("operation"), 11:w382) -> (3:w371:refnum<k34>)  [unwired: 4 in, 1 out]
        n177 = for {
          tunnel: w369 -> [w407] mode=indexing
          tunnel: w368 -> [w408]
          tunnel: [w406] -> w367 mode=indexing
          n178 = Equal?(x=w407, y=w408) -> (x = y?=w406:bool)
        }
        n179 = Bundle By Name(cluster=T20 {"recording?"=FALSE, "tdms file"=refnum} ("output cluster"), "tdms file"=w371, "recording?"="Recording?") -> (w386:T20)
        n180 = Or Array Elements(Boolean array=w367) -> (logical OR=w366:bool)
        "friction test?" <- w366
        n181 = Tick Count (ms)() -> (millisecond timer value=w395:u32)
        n182 = To Quad Integer(1:w395) -> (0:w394:i64)
        n183 = To Variant(anything=w386) -> (Variant=w390:variant)
        n184 = Negate(x=w394) -> (-x=w393:i64)
        n185 = Bundle By Name(cluster=cluster{"STATE":T18, "Data":variant} {"STATE"=enum."READY", "Data"=variant} ("element"), "Data"=w390) -> (w388:cluster{"STATE":T18, "Data":variant})
        n186 = Enqueue Element(queue=w392, element=w388, error in (no error)=w405) -> (error out=w404:errorcluster)  [unwired: 1 in, 2 out]
        n187 = To Variant(anything=w386) -> (Variant=w396:variant)
        n188 = Bundle By Name(cluster=cluster{"STATE":T19, "Data":variant} {"STATE"=enum."READY", "Data"=variant} ("element"), "Data"=w396) -> (w397:cluster{"STATE":T19, "Data":variant})
        n189 = Enqueue Element(queue=w391, element=w397, error in (no error)=w404) -> (error out=w402:errorcluster)  [unwired: 1 in, 2 out]
        n190 = Bundle By Name(cluster=w364, "PreTrialInfo"=w372, "friction test?"=w366, "TrialInfo"=w370, "dCOP cond"=w375, "state"=ctlTrialState."ready", "tick ini"=w393, "tdms data"=w371, "Recording?"="Recording?") -> (w403:T11)
      }
      frame "RepeatTrial" {
        n191 = Unbundle By Name(w410) -> ("PreTrialInfo"=w409:T14)
        n192 = Bundle By Name(cluster=w410, "TrialInfo"=w409) -> (w411:T11)
      }
      frame "Events" {
        n193 = Unbundle By Name(w413) -> ("dCOP cond"=w418:T7, "friction test?"=w417:bool, "state"=w435:T10, "PhaseSpace"=w419:refnum<queue>, "ATI"=w420:refnum<queue>, "Trigger Task"=w416:refnum<k21>)
        n194 = case shown="\"hold\"" w435 {
          selector: w435 -> [w450 w453 w458 w463 w466 w469]
          tunnel: [w450 w453 w458 w463 w466 w469] -> w437
          tunnel: ["" ("name or relative path") "ready" ("name or relative path") w456 "hold" ("name or relative path") "relax" ("name or relative path") "" ("name or relative path")] -> w427
          tunnel: w418 -> [_ _ w457 _ _ _]
          tunnel: w417 -> [_ _ w455 _ _ _]
          tunnel: [u8 8 u8 1 u8 2 u8 4 u8 8 u8 8] -> w415
          frame "no events", Default {
            # "This case should not be executed!"
          }
          frame "ready" {
          }
          frame "start" {
            n195 = case shown="True" w455 {
              tunnel: w457 -> [_ _]
              tunnel: ["go" ("name or relative path") "relax" ("name or relative path")] -> w456
              frame False {
              }
              frame True {
              }
            }
          }
          frame "hold" {
          }
          frame "stop" {
          }
          frame "end" {
          }
        }
        n196 = To Variant(anything=w437) -> (Variant=w436:variant)
        n197 = Build Array(w415) -> (w414:u8[])
        n198 = Bundle By Name(cluster=cluster{"STATE":T18, "Data":variant} {"STATE"=enum."TRIGGER", "Data"=variant} ("element"), "Data"=w436) -> (w438:cluster{"STATE":T18, "Data":variant})
        n199 = Bundle By Name(cluster=cluster{"STATE":T19, "Data":variant} {"STATE"=enum."TRIGGER", "Data"=variant} ("element"), "Data"=w436) -> (w439:cluster{"STATE":T19, "Data":variant})
        n200 = call <vilib>:"Application Directory.vi"() -> ("Application Directory"=w429:path)
        n201 = Enqueue Element At Opposite End(queue=w419, element=w439) -> (error out=w433:errorcluster)  [unwired: 2 in, 2 out]
        n202 = Enqueue Element At Opposite End(queue=w420, element=w438, error in (no error)=w424) -> (error out=w434:errorcluster)  [unwired: 1 in, 2 out]
        n203 = Build Path(base path=w429, name or relative path="audio cues") -> (appended path=w426:path)
        n204 = Concatenate Strings(w427, ".wav" ("name or relative path")) -> (w425:string)
        n205 = call-poly <vilib>:"DAQmx Write.vi"("task/channels in"=w416, "data"=w414) -> ()  [unwired: 11 in, 3 out]
        n206 = Merge Errors(w433, w434) -> (w431:errorcluster)
        n207 = Build Path(base path=w426, name or relative path=w425) -> (appended path=w423:path)
        n208 = call <vilib>:"Check if File or Folder Exists.vi"("path"=w423) -> ("file or folder exists?"=w421:bool, "dup path"=w422:path)  [unwired: 8 in, 1 out]
        n209 = case shown="True" w421 {
          tunnel: [w442 w445] -> w432
          tunnel: w431 -> [w442 w444]
          tunnel: w422 -> [_ w443]
          frame False {
          }
          frame True {
            n210 = call <vilib>:"Sound File Read Simple.vi"("error in (no error)"=w444, "path"=w443) -> ("error out"=w446:errorcluster, "data"=w447:waveform(dbl)[])  [unwired: 6 in, 2 out]
            n211 = call "Play Waveform"("Data"=w447, "error in"=w446) -> ("error out"=w445:errorcluster)  [unwired: 17 in]
          }
        }
      }
      frame "Get PhaseSpace" {
        w489 = T21 0 items=["X-Y-Z", "X-Z-Y", "Y-X-Z", "Y-Z-X", "Z-X-Y", "Z-Y-X", "X-Y-X", "X-Z-X", "Y-X-Y", "Y-Z-Y", "Z-X-Z", "Z-Y-Z"] ("roll-yaw-pitch")
        n212 = Unbundle By Name(w487) -> ("d2plane.frame"=w502:dbl[][])
        n213 = Variant To Data(error in=w508, type=T12[] [] ("Markers"), Variant=w510) -> (data=w472:T12[], error out=w507:errorcluster)
        n214 = Array Subset(array=w472, length=4) -> (w504:T12[])  [unwired: 1 in]
        n215 = Transpose 2D Array(2D array=w502) -> (transposed array=w501:dbl[][])
        n216 = call "GetFrame(SubVI).vi"("pt"=w504) -> ("frame [R T]"=w503:dbl[][])
        n217 = Delete From Array(array=w501) -> (deleted portion=w496:dbl[], array with subset deleted=w500:dbl[][])  [unwired: 3 in]
        n218 = Transpose 2D Array(2D array=w503) -> (transposed array=w498:dbl[][])
        n219 = Delete From Array(array=w498) -> (deleted portion=w495:dbl[], array with subset deleted=w499:dbl[][])  [unwired: 3 in]
        n220 = call-poly <vilib>:"Array To Matrix.vi"("Real 2D Array"=w500) -> ("Real Matrix"=w471:T22)
        n221 = Unbundle By Name(w487) -> ("maxroll"=w480:dbl, "maxheight"=w478:dbl)
        n222 = Transpose 2D Array(2D array=w499) -> (transposed array=w497:dbl[][])
        n223 = Subtract(x=w495, y=w496) -> (x-y=w476:dbl[])
        n224 = call-poly <vilib>:"Array To Matrix.vi"("Real 2D Array"=w497) -> ("Real Matrix"=w490:T22)
        n225 = Transpose Matrix(1:w471) -> (0:w475:T22)
        n226 = call-poly <vilib>:"A x B.vi"("B"=w471, "A"=w490) -> ("A x B"=w493:T22)  [unwired: 1 out]
        n227 = call-poly <vilib>:"Matrix To Array.vi"("Real Matrix"=w493) -> ("Real 2D Array"=w492:dbl[][])
        n228 = call-poly <vilib>:"A x B.vi"("Vector"=w476, "A"=w475) -> ("A x Vector"=w474:dbl[])  [unwired: 1 out]
        n229 = call <vilib>:"Direction Cosines To Euler Angles.vi"("rotation order"=w489, "Direction Cosines"=w492) -> ("Euler Angles"=w491:cluster{"phi":dbl, "theta":dbl, "psi":dbl})  [unwired: 8 in, 1 out]
        n230 = Index Array "Index Array"(array=w474, index=1) -> (element=w473:dbl)
        "h (mm)" <- w473
        n231 = expression code="(x/pi)*180.0" ("radians to degrees")(w491) -> (w488:cluster{"phi":dbl, "theta":dbl, "psi":dbl})
        n232 = Unbundle By Name(w488) -> ("phi"=w479:dbl)
        "Roll (deg)" <- w479
        n233 = Absolute Value(x=w473) -> (abs(x)=w486:dbl)
        n234 = Absolute Value(x=w478) -> (abs(x)=w484:dbl)
        n235 = Greater?(x=w486, y=w484) -> (0:w482:bool)
        n236 = Select(t=w473, s=w482, f=w478) -> (s? t:f=w477:dbl)
        "max height" <- w477
        n237 = Absolute Value(x=w479) -> (abs(x)=w481:dbl)
        n238 = Absolute Value(x=w480) -> (abs(x)=w485:dbl)
        n239 = Greater?(x=w481, y=w485) -> (0:w483:bool)
        n240 = Select(t=w479, s=w483, f=w480) -> (s? t:f=w470:dbl)
        "max roll" <- w470
        "Meter" <- w470
        n241 = Bundle By Name(cluster=w487, "Handle Tilt"=w479, "Handle Height"=w473, "maxroll"=w470, "maxheight"=w477, "Markers"=w472) -> (w506:T11)
      }
      frame "Get PS bias" {
        n242 = Variant To Data(error in=w516, type=T13 {"frame"=[]}, Variant=w517) -> (data=w512:T13, error out=w515:errorcluster)
        n243 = Bundle By Name(cluster=w514, "d2plane"=w512) -> (w513:T11)
      }
      frame "Get ATI" {
        w559 = -2.0
        w570 = -2.0
        # "Manipulation and Grasp Forces Decomposition"
        # "copy = -my/fz"
        # "copxIN = -mx/fz"
        # "copxTH = mx/fz"
        # "copy = -my/fz"
        n244 = Variant To Data(error in=w592, type=cluster{dbl[][]}[] [] ("Data"), Variant=w593) -> (data=w573:cluster{dbl[][]}[], error out=w591:errorcluster)
        "ATI" <- w573
        n245 = Bundle By Name(cluster=w589, "ATI Data"=w573) -> (w588:T11)
        n246 = Index Array(array=w573) -> (element #1=w587:cluster{dbl[][]}, element #2=w586:cluster{dbl[][]})  [unwired: 2 in]
        n247 = Unbundle(w587) -> (w585:dbl[][])
        n248 = Unbundle(w586) -> (w584:dbl[][])
        n249 = Delete From Array(array=w585) -> (deleted portion=w572:dbl[])  [unwired: 3 in, 1 out]
        n250 = Delete From Array(array=w584) -> (deleted portion=w571:dbl[])  [unwired: 3 in, 1 out]
        n251 = Build Array (concatenate)(w572, w571) -> (w582:dbl[])
        n252 = call "GraspMapTHIN_sensorFrame.vi"() -> ("Grasp Map"=w583:T22)
        n253 = call-poly <vilib>:"Array To Matrix.vi"("Real 1D Array"=w582) -> ("Real Matrix (Column Vector)"=w581:T22)
        n254 = call-poly <vilib>:"A x B.vi"("B"=w581, "A"=w583) -> ("A x B"=w578:T22)  [unwired: 1 out]
        n255 = Transpose 2D Array(2D array=w578) -> (transposed array=w574:T22)
        n256 = Index Array(array=w574) -> (element=w575:dbl[])  [unwired: 2 in]
        n257 = Index Array(array=w575) -> (element #4=w577:dbl, element #5=→"My":dbl)  [unwired: 6 in, 4 out]
        n258 = Index Array(array=w572, index #1=2 ("index"), index #2=3 ("index"), index #3=4 ("index")) -> (element #1=w561:dbl, element #2=w556:dbl, element #3=w551:dbl)
        n259 = Index Array(array=w571, index #1=2 ("index"), index #2=3 ("index"), index #3=4 ("index")) -> (element #1=w565:dbl, element #2=w567:dbl, element #3=w544:dbl)
        n260 = Less?(x=w559, y=w561) -> (x < y?=w558:bool)
        n261 = Less?(x=w570, y=w565) -> (x < y?=w569:bool)
        n262 = Index Array(array=w572, index #1=0 ("index"), index #2=1 ("index"), index #3=2 ("index"), index #4=5 ("index")) -> (element #1=w538:dbl, element #2=w537:dbl, element #3=w536:dbl, element #4=w535:dbl)
        n263 = Multiply(x=w577, y=1000.0) -> (x*y=→"Mx":dbl)
        n264 = Select(t=w559, s=w558, f=w561) -> (s? t:f=w557:dbl)
        n265 = Select(t=w570, s=w569, f=w565) -> (s? t:f=w568:dbl)
        n266 = Reciprocal(x=w557) -> (1/x=w552:dbl)
        n267 = Reciprocal(x=w568) -> (1/x=w545:dbl)
        n268 = Compound Arithmetic op=MULTIPLY(w552, w556) -> (w554:dbl)
        n269 = Index Array(array=w571, index #1=0 ("index"), index #2=1 ("index"), index #3=2 ("index"), index #4=5 ("index")) -> (element #1=w530:dbl, element #2=w529:dbl, element #3=w528:dbl, element #4=w527:dbl)
        n270 = Compound Arithmetic op=MULTIPLY(w552, w551) -> (w563:dbl)
        n271 = Compound Arithmetic op=MULTIPLY(w545, w567) -> (w564:dbl)
        n272 = Compound Arithmetic op=MULTIPLY(w545, w544) -> (w547:dbl)
        n273 = Negate(x=w563) -> (-x=w562:dbl)
        n274 = Negate(x=w564) -> (-x=w548:dbl)
        n275 = Negate(x=w547) -> (-x=w546:dbl)
        n276 = Build Array(w538, w537, w536, w535, w530, w529, w528, w527) -> (w524:dbl[])
        n277 = call "GraspMapTHIN.vi"("copyIN (m)"=w546, "copxIN (m)"=w548, "copyTH (m)"=w562, "copxTH (m)"=w554) -> ("Grasp Map"=w519:T22)
        n278 = call "FindNullSpace (SubVI).vi"("Matrix"=w519) -> ("Null"=w518:T22)  [unwired: 1 out]
        n279 = Transpose 2D Array(2D array=w518) -> (transposed array=w543:T22)
        n280 = call-poly <vilib>:"A x B.vi"("B"=w543, "A"=w518) -> ("A x B"=w526:T22)  [unwired: 1 out]
        n281 = call-poly <vilib>:"A x B.vi"("Vector"=w524, "A"=w526) -> ("A x Vector"=w523:dbl[])  [unwired: 1 out]
        "FG" <- w523
        n282 = Negate(x=w523) -> (-x=w525:dbl[])
        n283 = call-poly <vilib>:"Vector Norm.vi"("Input Vector"=w523) -> ("norm"=→"|FG| (N)":dbl)  [unwired: 9 in, 1 out]
        n284 = Add(x=w525, y=w524) -> (x+y=w522:dbl[])
        "FM" <- w522
        n285 = call-poly <vilib>:"Vector Norm.vi"("Input Vector"=w522) -> ("norm"=→"|FM| (N)":dbl)  [unwired: 9 in, 1 out]
      }
      frame "Finish" {
        n286 = Unbundle By Name(w599) -> ("Trigger Task"=w594:refnum<k21>, "PhaseSpace"=w606:refnum<queue>, "ATI"=w605:refnum<queue>)
        n287 = Enqueue Element(queue=w605, element=cluster{"STATE":T18, "Data":variant} {"STATE"=enum."END", "Data"=variant}, error in (no error)=w608) -> (error out=w607:errorcluster)  [unwired: 1 in, 2 out]
        n288 = Bundle By Name(cluster=w599, "state"=ctlTrialState."no events", "Markers"=T12[] [], "ATI Data"=cluster{dbl[][]}[] [] ("Data")) -> (w597:T11)
        n289 = Enqueue Element(queue=w606, element=cluster{"STATE":T19, "Data":variant} {"STATE"=enum."END", "Data"=variant}, error in (no error)=w607) -> (error out=w598:errorcluster)  [unwired: 1 in, 2 out]
        n290 = disable-structure shown="Disabled" {
          frame Disabled {
            n291 = Select(t=T15."Enabled" ("Disabled"), f=T15."Disabled and Grayed Out" ("Disabled")) -> (s? t:f=w611:T15)  [unwired: 1 in]
            n292 = property on="Ready" class="Bool"("DisabledEnum"=w611) -> ()  [unwired: 2 in, 2 out]
          }
          frame Enabled {
          }
        }
        n293 = call-poly <vilib>:"DAQmx Write.vi"("task/channels in"=w594, "data"=u8[] [0]) -> ()  [unwired: 11 in, 3 out]
        n294 = property on="Bias" class="Bool"("DisabledEnum"=T15."Enabled" ("Disabled")) -> ()  [unwired: 2 in, 2 out]
      }
      frame "End PhaseSpace" {
        n295 = Bundle By Name(cluster=w615, "PhaseSpace end?"=TRUE) -> (w614:T11)
      }
      frame "End ATI" {
        n296 = Bundle By Name(cluster=w619, "ATI end?"=TRUE ("PhaseSpace end?")) -> (w618:T11)
      }
      frame "ERROR" {
        # "Error Dialog"
        # "Error is cleared after handling"
        n297 = call <vilib>:"Simple Error Handler.vi"("error in (no error)"=w621) -> ()  [unwired: 4 in, 5 out]
        n298 = call "Error Clear.vi"("error in"=w621) -> ("error in (no error)"=w620:errorcluster)  [unwired: 7 in]
      }
      frame "EXIT" {
        # "Sending exit command to parallel processes"
        n299 = global write "GLOBAL -MAIN.vi" "EXIT"(TRUE ("EXIT")) -> ()
        n300 = Unbundle By Name(w632) -> ("PhaseSpace"=w631:refnum<queue>, "ATI"=w630:refnum<queue>, "Trigger Task"=w624:refnum<k21>)
        n301 = call <vilib>:"DAQmx Clear Task.vi"("task in"=w624) -> ()  [unwired: 14 in, 1 out]
        n302 = Enqueue Element(queue=w630, element=cluster{"STATE":T18, "Data":variant} {"STATE"=enum."EXIT", "Data"=variant}, error in (no error)=w625) -> (error out=w633:errorcluster)  [unwired: 1 in, 2 out]
        n303 = Enqueue Element(queue=w631, element=cluster{"STATE":T19, "Data":variant} {"STATE"=enum."EXIT", "Data"=variant}, error in (no error)=w633) -> (error out=w623:errorcluster)  [unwired: 1 in, 2 out]
        n304 = property on="STOP" class="Bool"(error in=w623, "DisabledEnum"=T15."Enabled" ("Disabled")) -> (error out=w627:errorcluster)  [unwired: 1 in, 1 out]
      }
    }
    n305 = call "STTM Q MGR.vi"("QSTATES"=w13, "QRef"=w12, "Error IN"=w20, "FNs"=w14) -> ("Error OUT"=w19:errorcluster)  [unwired: 11 in]
  }
  n306 = while "Events" {
    tunnel: 150 -> [w639]
    tunnel: w4 -> [_]
    tunnel: w2 -> [w635]
    stop <- w636 stop-if-true
    n307 = event shown="[6] \"Path\": Value Change" {
      selector: _ -> [_ _ _ _ _ _ _ _]
      dyn-events: _ -> [_ _ _ _ _ _ _ _]
      timeout: w639 -> [_ _ _ _ _ _ _ _]
      tunnel: [FALSE _ _ _ _ _ _ _] -> w638
      tunnel: w635 -> [_ w643 w645 w648 w655 w661 w666 w670]
      event Timeout {
        n308 = event-data() -> ()  [unwired: 1 in, 1 out]
      }
      event "Ready": Value Change {
        w641 = T15."Disabled and Grayed Out" ("Disabled")
        # "Producer event case adding send message command"
        n309 = event-data() -> ()  [unwired: 1 in, 2 out]
        n310 = Enqueue Element(queue=w643, element=cluster{"STATE":T5, "Data":variant} {"STATE"=enum."Ready", "Data"=variant}) -> ()  [unwired: 2 in, 3 out]
        n311 = property on="Ready" class="Bool"("DisabledEnum"=w641) -> ()  [unwired: 2 in, 2 out]
        n312 = property on="Bias" class="Bool"("DisabledEnum"=w641) -> ()  [unwired: 2 in, 2 out]
      }
      event "RepeatTrial": Value Change {
        n313 = event-data() -> ()  [unwired: 1 in, 2 out]
        n314 = Enqueue Element(queue=w645, element=cluster{"STATE":T5, "Data":variant} {"STATE"=enum."RepeatTrial", "Data"=variant}) -> ()  [unwired: 2 in, 3 out]
      }
      event "Bias": Value Change {
        # "Producer event case adding send message command"
        n315 = event-data() -> ()  [unwired: 1 in, 2 out]
        n316 = Enqueue Element(queue=w648, element=cluster{"STATE":T5, "Data":variant} {"STATE"=enum."Bias", "Data"=variant}) -> ()  [unwired: 2 in, 3 out]
        n317 = property on="Ready" class="Bool"("DisabledEnum"=T15."Enabled" ("Disabled")) -> ()  [unwired: 2 in, 2 out]
      }
      event Value Change {
        w650 = T8 {"Subject ID"=enum."sub-00", "Block order"=[enum."RHP", enum."RLD", enum."RHD", enum."LHP", enum."LLD", enum."LHD", enum."UR", enum."UL", enum."pstDrop", enum."famDrop", enum."famDrop", enum."famDrop"]}  # InitializeProtocol
        n318 = event-data() -> ()  [unwired: 1 in, 1 out]
        n319 = Bundle By Name(cluster=w650, "Subject ID"="Subject ID") -> (w649:T8)
        n320 = To Variant(anything=w649) -> (Variant=w653:variant)
        n321 = Bundle By Name(cluster=cluster{"STATE":T5, "Data":variant} {"STATE"=enum."UpdateProtocol", "Data"=variant} ("element"), "Data"=w653) -> (w654:cluster{"STATE":T5, "Data":variant})
        n322 = Enqueue Element(queue=w655, element=w654) -> ()  [unwired: 2 in, 3 out]
        n323 = property on="Bias" class="Bool"("DisabledEnum"=T15."Enabled" ("Disabled")) -> ()  [unwired: 2 in, 2 out]
      }
      event Value Change {
        n324 = event-data() -> ()  [unwired: 1 in, 1 out]
        n325 = To Variant(anything="BlockInfoSet") -> (Variant=w659:variant)
        n326 = Bundle By Name(cluster=cluster{"STATE":T5, "Data":variant} {"STATE"=enum."UpdateBlockInfo", "Data"=variant} ("element"), "Data"=w659) -> (w660:cluster{"STATE":T5, "Data":variant})
        n327 = Enqueue Element(queue=w661, element=w660) -> ()  [unwired: 2 in, 3 out]
        n328 = property on="Bias" class="Bool"("DisabledEnum"=T15."Enabled" ("Disabled")) -> ()  [unwired: 2 in, 2 out]
      }
      event "Path": Value Change {
        n329 = event-data() -> ()  [unwired: 1 in, 1 out]
        n330 = To Variant(anything="Path") -> (Variant=w664:variant)
        n331 = Bundle By Name(cluster=cluster{"STATE":T5, "Data":variant} {"STATE"=enum."UpdatePath", "Data"=variant} ("element"), "Data"=w664) -> (w665:cluster{"STATE":T5, "Data":variant})
        n332 = Enqueue Element(queue=w666, element=w665) -> ()  [unwired: 2 in, 3 out]
      }
      event "STOP": Value Change {
        w668 = T15."Disabled and Grayed Out" ("Disabled")
        # "Producer event case adding exit command"
        n333 = event-data() -> ()  [unwired: 1 in, 3 out]
        n334 = Enqueue Element(queue=w670, element=cluster{"STATE":T5, "Data":variant} {"STATE"=enum."EXIT", "Data"=variant}) -> ()  [unwired: 2 in, 3 out]
        n335 = property on="Ready" class="Bool"("DisabledEnum"=w668) -> ()  [unwired: 2 in, 2 out]
        n336 = property on="STOP" class="Bool"("DisabledEnum"=w668) -> ()  [unwired: 2 in, 2 out]
      }
    }
    n337 = global read "GLOBAL -MAIN.vi" "EXIT"() -> (w637:bool)
    n338 = Or(x=w638, y=w637) -> (x .or. y?=w636:bool)
  }
  n339 = flat-sequence {
    tunnel: w4 -> [_]
    frame #0 {
      # "Parallel processes which themselves are both consumer producer processes"
      n340 = call "SubVI PhaseSpace.vi"() -> ()  [unwired: 16 in]
      n341 = call "SubVI ATI.vi"() -> ()  [unwired: 16 in]
    }
  }
  n342 = Release Queue(queue=w9, force destroy? (F)=TRUE) -> ()  [unwired: 1 in, 3 out]
